vi "Pi-Drive (SubVI).vi"(9 "Turn":dbl, 10 "Throttle":dbl) -> (2 "Right Drive":dbl, 3 "Left Drive":dbl)   [LabVIEW 2017]
panel:
  in  "QuickTurn Gain":dbl=0.6 format="%#_13g"
  in  "Throttle Deadband":dbl=0.1
  # "Inputs"
  # "Controls"
  # "Outputs"
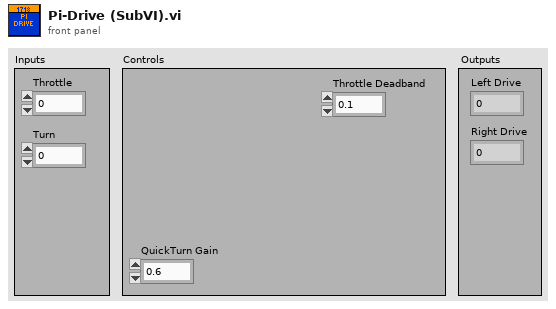
[diagram p1: front panel]
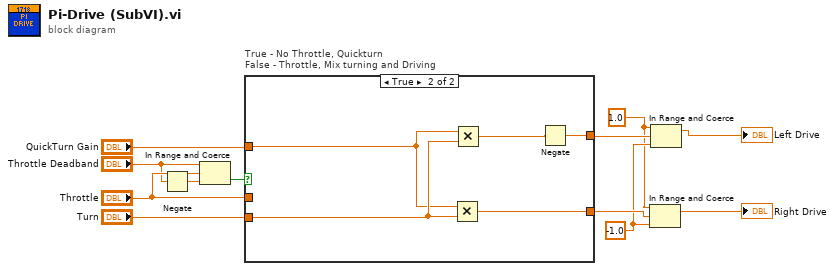
[diagram p0: block diagram]
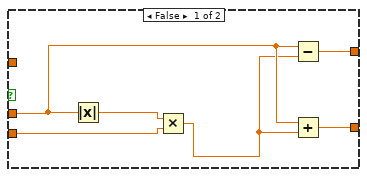
[diagram p2: hidden frame]
diagram:
  w3 = -1.0 ("lower limit")
  w2 = 1.0 ("upper limit")
  n1 = Negate(x="Throttle Deadband") -> (-x=w9:dbl)
  n2 = In Range and Coerce(upper limit="Throttle Deadband", x="Throttle", lower limit=w9) -> (In Range?=w8:bool)  [unwired: 1 out]
  n3 = case "True - No Throttle, Quickturn\nFalse - Throttle, Mix turning and Driving" shown="True" w8 {
    tunnel: "Turn" -> [w14 w23]
    tunnel: [w17 w19] -> w7
    tunnel: [w18 w21] -> w6
    tunnel: "Throttle" -> [w15 _]
    tunnel: "QuickTurn Gain" -> [_ w22]
    frame False {
      n4 = Absolute Value(x=w15) -> (abs(x)=w16:dbl)
      n5 = Multiply(x=w16, y=w14) -> (x*y=w13:dbl)
      n6 = Subtract(x=w15, y=w13) -> (x-y=w18:dbl)
      n7 = Add(x=w15, y=w13) -> (x+y=w17:dbl)
    }
    frame True {
      n8 = Multiply(x=w22, y=w23) -> (x*y=w19:dbl)
      n9 = Multiply(x=w22, y=w23) -> (x*y=w20:dbl)
      n10 = Negate(x=w20) -> (-x=w21:dbl)
    }
  }
  n11 = In Range and Coerce(upper limit=w2, x=w7, lower limit=w3) -> (coerced(x)=→"Right Drive":dbl)  [unwired: 1 out]
  n12 = In Range and Coerce(upper limit=w2, x=w6, lower limit=w3) -> (coerced(x)=→"Left Drive":dbl)  [unwired: 1 out]
